vi "Write Status.vi"(8 "error in (no error)":errorcluster, 10 "Status Bitfield":u16, 11 "Storage Line in":refnum<class "Storage Line.lvclass">) -> (0 "error out":errorcluster, 2 "Status Bitfield":u16, 3 "Storage Line out":refnum<class "Storage Line.lvclass">)   [LabVIEW 2015, in "cRIO-Carbondioxide.lvlib" / "CO2-Actor.lvlib" / "Storage Line.lvclass"]
uses:
  Storage Line.lvclass
  Storage Line.lvclass/Storage Line.ctl
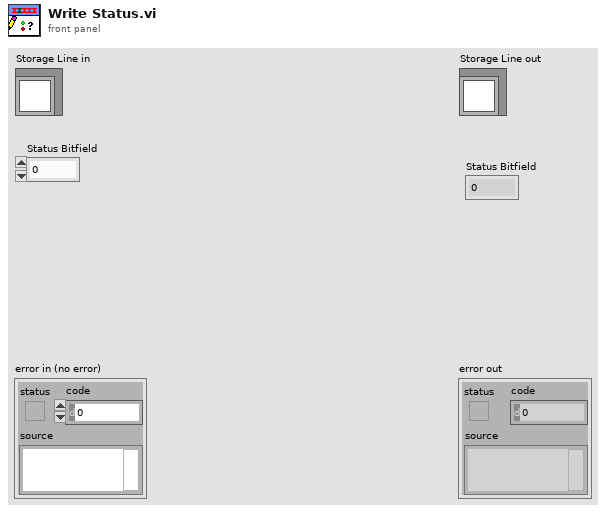
[diagram p1: front panel]
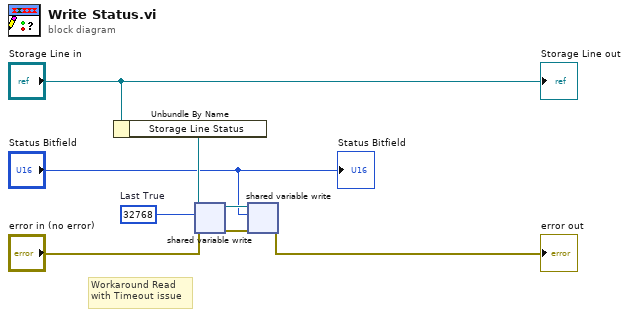
[diagram p0: block diagram]
diagram:
  w4 = u16 32768  # Last True
  # "Workaround Read \nwith Timeout issue"
  n1 = Unbundle By Name("Storage Line in") -> ("Storage Line Status"=w7:refnum<k21>)
  n2 = shared-variable-write(w7, "error in (no error)", w4) -> (w5:refnum<k21>, w6:errorcluster)
  n3 = shared-variable-write(w5, w6, "Status Bitfield") -> (→"error out":errorcluster)  [unwired: 1 out]
  "Storage Line out" <- "Storage Line in"
  "Status Bitfield" <- "Status Bitfield"
